vi "AKD Stop.vi"(0 "connection ID":refnum<k5>, 11 "error in":errorcluster) -> (4 "TCP Refnum":refnum<k5>, 15 "error out":errorcluster)   [LabVIEW 2024]
uses:
  MODBUS/NI Modbus.llb/MB Ethernet Master Query Write Multiple Registers (poly).vi
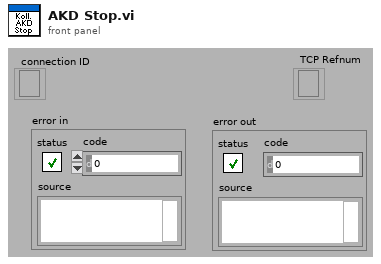
[diagram p1: front panel]
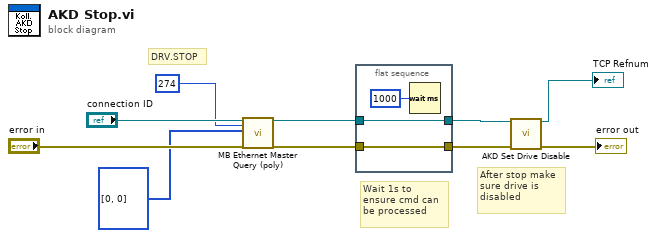
[diagram p0: block diagram]
diagram:
  # "Wait 1s to \nensure cmd can\nbe processed"
  # "After stop make\nsure drive is \ndisabled"
  # "DRV.STOP"
  n1 = call-poly "MB Ethernet Master Query (poly).vi"("TCP Connection Refnum in"="connection ID", "Starting Address"=u16 274, "Registers"=u16[] [0, 0], "error in"="error in") -> ("TCP Connection Refnum (dup)"=w3:refnum<k5>, "error out"=w2:errorcluster)  [unwired: 13 in, 1 out]
  n2 = flat-sequence {
    tunnel: [w12] -> w4
    tunnel: w3 -> [w12]
    tunnel: w2 -> [w11]
    tunnel: [w11] -> w1
    frame #0 {
      n3 = Wait (ms)(milliseconds to wait=u32 1000) -> ()  [unwired: 1 out]
    }
  }
  n4 = call "AKD Set Drive Disable.vi"("connection ID"=w4, "error in"=w1) -> ("TCP Refnum"=→"TCP Refnum":refnum<k5>, "error out"=→"error out":errorcluster)  [unwired: 12 in]
